vi "main.vi"() -> ()   [LabVIEW 2019]
panel:
  in  "Control Tab":T1(tab)
  out "Error Consumer":errorcluster
  out "Error Producer":errorcluster
  out "Error Close":errorcluster
  out "Error GUI":errorcluster
  out "Error Message Generator":errorcluster
  out "VI Description":string
  out "VI-filename":string
  out "VI Path":path
  out "Code Size":u32
  out "Revision Number":u32
  in  "Tool Bar:Visible":bool
  out "Application Name":string
  out "Project name":string
  out "Description":string
  out "Path":path
  out "VI-Name":string
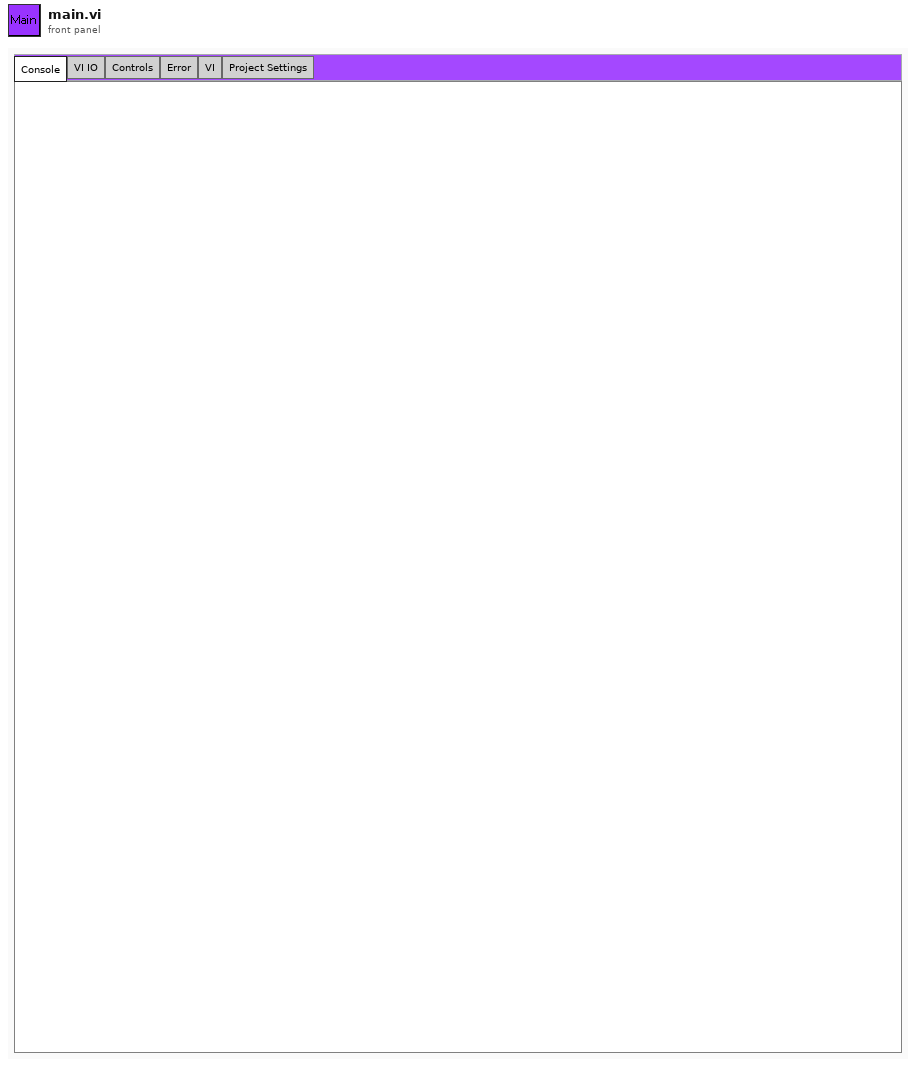
[diagram p1: front panel]
types:
  T1 = enum32{"Console", "VI IO", "Controls", "Error", "VI", "Project Settings"}
  T2 = enum32{"Invalid", "Standard", "Closed", "Hidden", "Minimized", "Maximized"}
  T3 = typedef "Application_Data.ctl" = cluster{"Console log":string, "GUI_Events":T4, "Function_Queue":T5, "Timout-Time[ms]":i32, "MIDI-Messages":T6, "Com Session State":T9, "Result Data":T10, "Get #":bool[], "CPU(ms)":u32}
  T4 = typedef "App_Events.ctl" = cluster{"To_GUI-Producer":refnum<user-event>, "To_GUI-Error_message":refnum<user-event>, "To_GUI-msg_list":refnum<user-event>, "To_GUI-Session":refnum<user-event>, "To_GUI-Pre-Session":refnum<user-event>, "To_GUI-Consumer":refnum<user-event>}
  T5 = typedef "App_Queues.ctl" = cluster{"Queue_MIDI_Handler":refnum<queue>, "Queue_Session":refnum<queue>, "Queue_Producer":refnum<queue>, "Queue_Consumer":refnum<queue>}
  T6 = typedef "MIDI-Message_Array.ctl" = T7[]
  T7 = typedef "MIDI-Message_Cluster.ctl" = cluster{"Message Name":string, "Meta value":i32, "Datastring":string, "Datatype":T8}
  T8 = typedef "Meta_Commands.ctl" = enum16{"No Data", "Pause", "Loop", "Wait for Rx", "Delay", "Break", "MIDI"}
  T9 = typedef "Session_State.ctl" = enum16{"Wait to begin", "Active Session", "Pause", "Wait for Response", "Stop", "Restart", "Inspect", "Exit"}
  T10 = typedef "Consumer_Result.ctl" = cluster{"Diff":bool[], "Tx Byte":string[], "Rx Byte":string[], "Send Log":string[], "Parsed Data":T11}
  T11 = typedef "Parsed_Data.ctl" = cluster{"Tx MIDI Tag":string[], "Tx MIDI Parsed Data":string[], "Tx Error":bool[], "Tx Running States":string[], "Rx MIDI Tag":string[], "Rx MIDI Parsed Data":string[], "Rx Error":bool[], "Rx Running States":string[], "Diff":bool[]}
  T12 = typedef "Producer-Data.ctl" = cluster{"Queue_Producer":refnum<queue>, "Queue_Consumer":refnum<queue>, "To_GUI-Error_message":refnum<user-event>, "Rx-Data":i8[], "Tx-Data":i8[], "Console log":string, "Communication Settings":T13, "MIDI-Messages":T6, "Queue_Session":refnum<queue>, "To_GUI-Pre-Session":refnum<user-event>, "To_GUI-Producer":refnum<user-event>, "Tx Info":T15, "Payload":variant, "Timout-Time[ms]":i32, "To_GUI-Session":refnum<user-event>, "CPU(ms)":u32}
  T13 = typedef "Communication_Settings.ctl" = cluster{"Tx Protocol":T14, "Rx Protocol":T14, "Serial":cluster{"Tx Port":refnum<visa-resource-name>, "Rx Port":refnum<visa-resource-name>, "Baud rate":i32, "Parity":enum16{"None", "Odd", "Even", "Mark", "Space"}, "Data bits":i32, "Stop bits":i32, "Flow control":enum16{"None", "XON/XOFF", "RTS/CTS", "XON/XOFF & RTS/CTS", "DTR/DSR", "XON/XOFF & DTR/DSR"}, "Tx Resource":refnum<visa-resource-name>, "Rx Resource":refnum<visa-resource-name>}, "MIDI Device":cluster{"Input uDevice ID":u32, "Output uDevice ID":u32, "hmidiout Handle":i32, "hmidiin Handle":i32}, "Bluetooth":cluster{"Dummy":string}, "USB":cluster{"Dummy":string}}
  T14 = typedef "Communication_Protocols.ctl" = enum16{"Serial", "Bluetooth", "USB-MIDI", "MIDI (Audio Device)", "Not Active"}
  T15 = typedef "Prod - Tx_Info.ctl" = cluster{"Datatype":T8[], "Bytesize":i32[], "Strings":string[], "ByteSum":i32}
  T16 = typedef "MIDI-Data.ctl" = cluster{"Console log":string, "Payload":variant, "MIDI Message Array":T6, "Timout-Time[ms]":i32, "Queue_MIDI_Handler":refnum<queue>, "To_GUI-Error_message":refnum<user-event>, "To_GUI-msg_list":refnum<user-event>, "CPU(ms)":u32}
  T17 = typedef "Consumer_Data.ctl" = cluster{"Queue_Consumer":refnum<queue>, "Selected Consumer":T18, "Session Data":T19, "Timout-Time[ms]":i32, "To_GUI-Consumer":refnum<user-event>, "CPU(ms)":u32, "Console log":string, "MIDI Parse Data":T20, "Session Inspection Data":T10}
  T18 = typedef "Consumer_States.ctl" = enum16{"Random", "ECG", "Strech-Patch"}
  T19 = typedef "Transfer_Data.ctl" = cluster{"Tx-Data":i8[], "Rx-Data":i8[], "MIDI-Message log":T6}
  T20 = typedef "Parser-data.ctl" = cluster{"MIDI-Bytes In":u8[], "MIDI Tag":string[], "MIDI Parsed Data":string[], "Iteration":i32, "Error?":bool[], "Running States":string[], "Running Statusbyte":u8, "Running StatusString":string, "Third Byte Flag":bool, "Current Byte":u8, "Sysex":string, "Expect Databyte":bool}
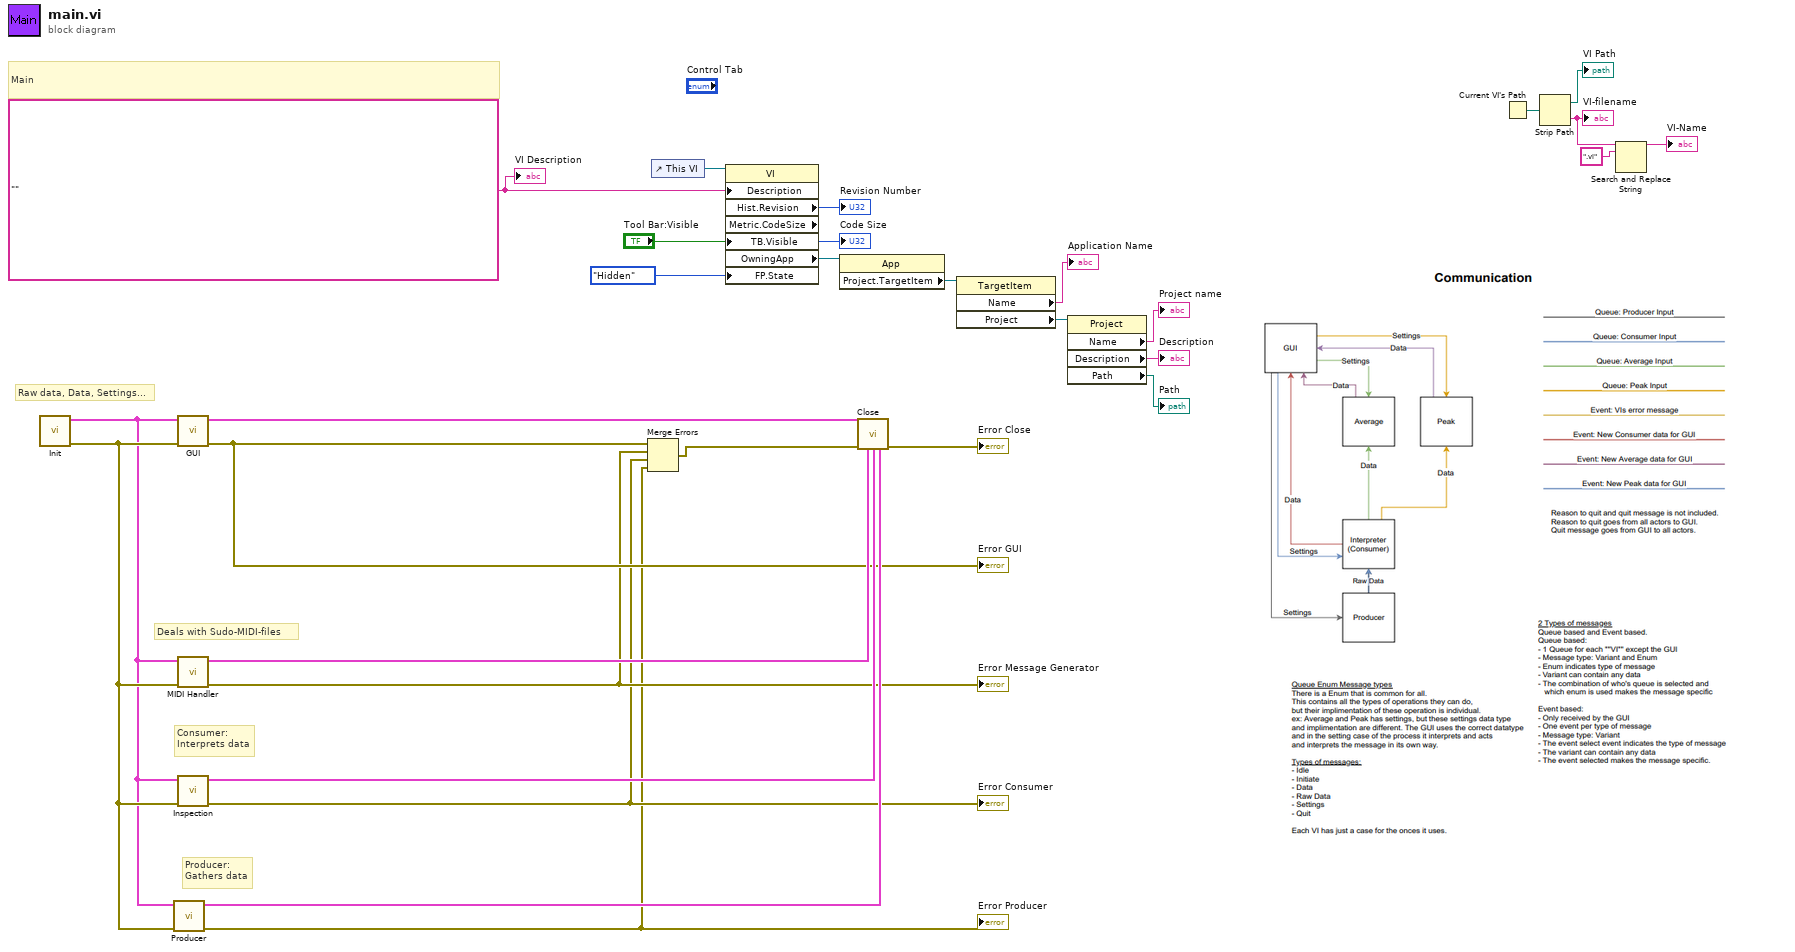
[diagram p0: block diagram]
diagram:
  w20 = ""
  # "Deals with Sudo-MIDI-files"
  # "Raw data, Data, Settings..."
  # "Consumer:\nInterprets data"
  # "Producer:\nGathers data"
  # "Main"
  n1 = call "Init.vi"() -> ("Error Out"=w11:errorcluster, "App Data Out"=w10:T3)  [unwired: 10 in]
  n2 = call "Producer.vi"("Error In"=w11, "App Data In"=w10) -> ("Error Out"=w2:errorcluster, "Producer-Data"=w6:T12)  [unwired: 8 in]
  "Error Producer" <- w2
  n3 = call "GUI.vi"("Error In"=w11, "Data in"=w10) -> ("Error Out"=w5:errorcluster, "Data out"=w28:T3)  [unwired: 8 in]
  "Error GUI" <- w5
  n4 = call "MIDI Handler.vi"("Error In"=w11, "App-Data In"=w10) -> ("Error Out"=w4:errorcluster, "MIDI Data Out"=w8:T16)  [unwired: 8 in]
  "Error Message Generator" <- w4
  n5 = call "Inspection.vi"("Error In"=w11, "Data In"=w10) -> ("Error Out"=w3:errorcluster, "Consumer Data"=w7:T17)  [unwired: 8 in]
  "Error Consumer" <- w3
  n6 = Merge Errors(w5, w4, w3, w2) -> (w1:errorcluster)
  n7 = control-ref of="This VI"() -> (w9:refnum<vi>)
  n8 = property class="VI"(reference=w9, "Description"=w20, "TB.Visible"="Tool Bar:Visible", "FP.State"=T2."Hidden" ("Front Panel Window:State")) -> ("Hist.Revision"=→"Revision Number":u32, "Metric.CodeSize"=→"Code Size":u32, "OwningApp"=w19:refnum<vi>)  [unwired: 1 in, 2 out]
  n9 = property class="App"(reference=w19) -> ("Project.TargetItem"=w18:refnum<vi>)  [unwired: 1 in, 2 out]
  n10 = call "Close.vi"("Data In"=w28, "Error In"=w1, "MIDI Data"=w8, "Consumer Data"=w7, "Producer-Data"=w6) -> ("Error Out"=→"Error Close":errorcluster)  [unwired: 10 in]
  n11 = property class="TargetItem"(reference=w18) -> ("Name"=→"Application Name":string, "Project"=w16:refnum<vi>)  [unwired: 1 in, 2 out]
  n12 = property class="Project"(reference=w16) -> ("Name"=→"Project name":string, "Description"=→"Description":string, "Path"=→"Path":path)  [unwired: 1 in, 2 out]
  n13 = Current VI's Path() -> (path=w30:path)
  n14 = Strip Path(path=w30) -> (stripped path=→"VI Path":path, name=w25:string)
  "VI-filename" <- w25
  n15 = Search and Replace String(input string=w25, search string=".vi") -> (result string=→"VI-Name":string)  [unwired: 6 in, 3 out]
  "VI Description" <- w20
